vi "Traverse Folder.vi"(5 "NEXT":bool, 7 "PREV":bool, 8 "error in (no error)":errorcluster, 10 "Context":T1, 11 "Boolean in":refnum<vi>) -> (0 "error out":errorcluster, 2 "Context out":T1)   [LabVIEW 2020, in "DocTool.lvlib"]
uses:
  DocTool.lvlib
  TDefs/Context.ctl
  Events.ctl
  UserEvent.ctl
  TDefs/State.ctl
  TDefs/States.ctl
  TDefs/Single File Properties.ctl
  TDefs/FP Items Properties.ctl
  TDefs/FP Item Properties.ctl
  TDefs/CopyTag.ctl
  d44677d1-7ccb-46bd-9aaf-ca2af3999deb.vi
  StateMachine.lvlib
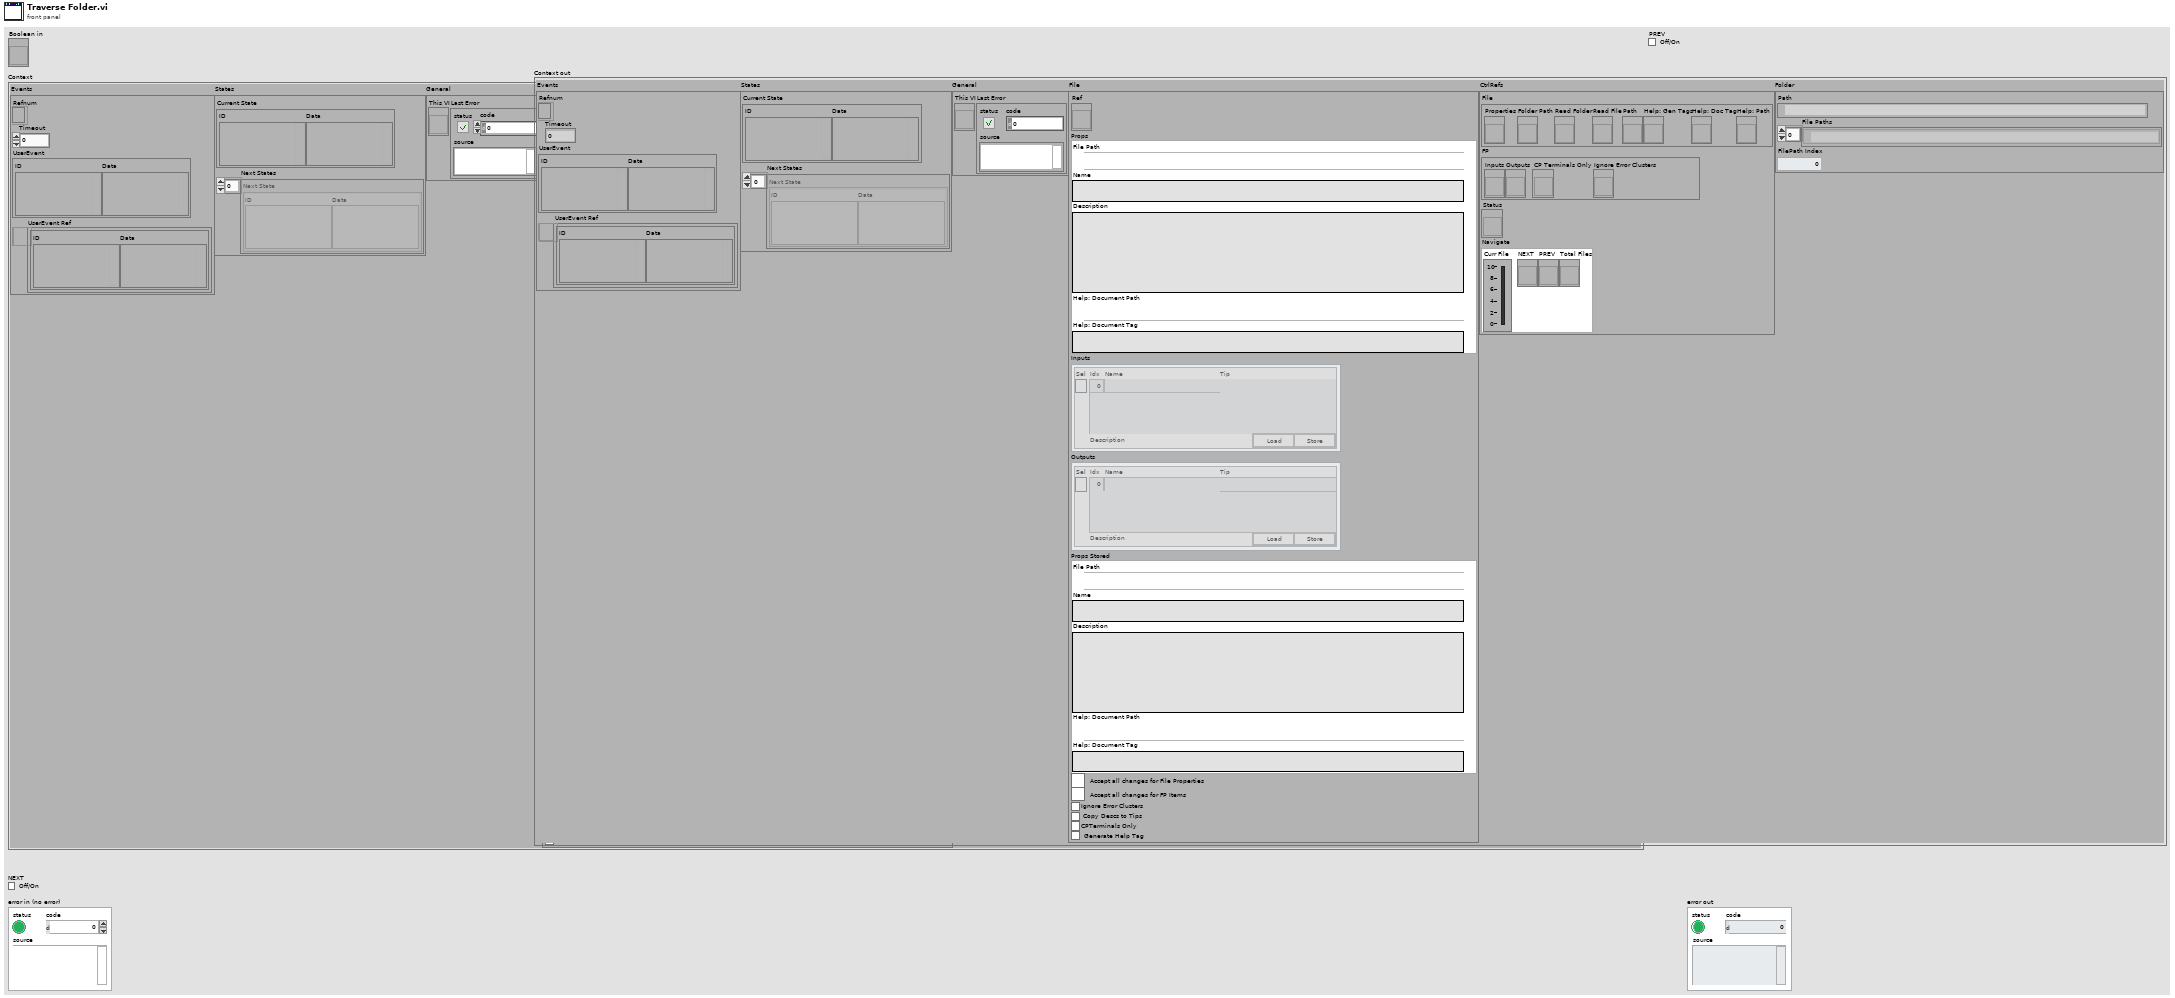
[diagram p1: front panel]
types:
  T1 = typedef "DocTool.lvlib/Context.ctl" = cluster{"Events":T2, "States":cluster{"Current State":T4, "Next States":T5}, "General":cluster{"This VI":refnum<vi>, "Last Error":errorcluster}, "File":cluster{"Ref":refnum<vi>, "Props":T6, "Inputs":T7, "Outputs":T7, "Props Stored":T6, "Write":bool, "Write FP":bool, "Ignore Error Clusters":bool, "Copy Descs to Tips":bool, "CPTerminals Only":bool, "Generate Help Tag":bool}, "CtrlRefs":cluster{"File":cluster{"Properties":refnum<vi>, "Folder Path":refnum<vi>, "Read Folder":refnum<vi>, "Read File":refnum<vi>, "Path":refnum<vi>, "Help: Gen Tags":refnum<vi>, "Help: Doc Tag":refnum<vi>, "Help: Path":refnum<vi>}, "FP":cluster{"Inputs":refnum<vi>, "Outputs":refnum<vi>, "CP Terminals Only":refnum<vi>, "Ignore Error Clusters":refnum<vi>}, "Status":refnum<vi>, "Navigate":cluster{"Curr File":refnum<vi>, "NEXT":refnum<vi>, "PREV":refnum<vi>, "Total Files":refnum<vi>}}, "Folder":cluster{"Path":path, "File Paths":path[], "FilePath Index":i32}}
  T2 = typedef "StateMachine.lvlib/Events.ctl" = cluster{"Refnum":refnum<event-registration>, "Timeout":i32, "UserEvent":T3, "UserEvent Ref":refnum<user-event>}
  T3 = typedef "StateMachine.lvlib/UserEvent.ctl" = cluster{"ID":variant, "Data":variant}
  T4 = typedef "StateMachine.lvlib/State.ctl" = cluster{"ID":variant, "Data":variant}
  T5 = typedef "StateMachine.lvlib/States.ctl" = T4[]
  T6 = typedef "DocTool.lvlib/Single File Properties.ctl" = cluster{"File Path":path, "Name":string, "Description":string, "Help: Document Path":path, "Help: Document Tag":string}
  T7 = typedef "DocTool.lvlib/FP Items Properties.ctl" = T8[]
  T8 = typedef "DocTool.lvlib/FP Item Properties.ctl" = cluster{"Sel":bool, "Idx":i32, "Name":string, "Description":string, "Tip":string, "Load Store":T9}
  T9 = typedef "DocTool.lvlib/CopyTag.ctl" = cluster{"Load":bool, "Store":bool}
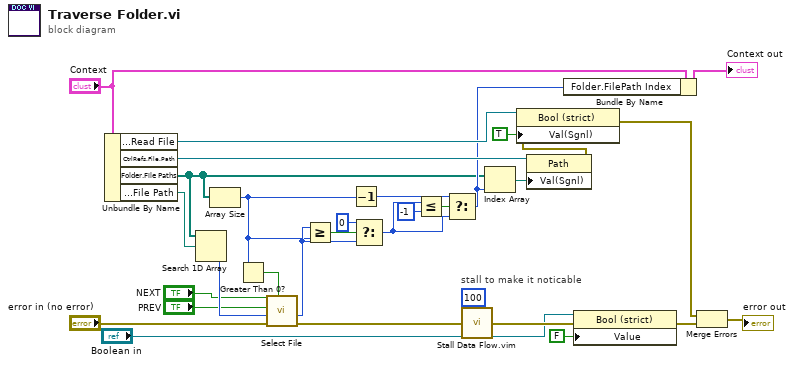
[diagram p0: block diagram]
diagram:
  # "stall to make it noticable"
  n1 = Unbundle By Name("Context") -> ("CtrlRefs.File.Read File"=w28:refnum<vi>, "CtrlRefs.File.Path"=w25:refnum<vi>, "Folder.File Paths"=w2:path[], "File.Props.File Path"=w26:path)
  n2 = Search 1D Array(1D array=w2, element=w26) -> (index of element=w27:i32)  [unwired: 1 in]
  n3 = Array Size(array=w2) -> (size(s)=w3:i32)
  n4 = Greater Than 0?(x=w3) -> (x > 0?=w6:bool)
  n5 = call "Select File.vi"("Files Found"=w6, "error in (no error)"="error in (no error)", "Current File in"=w27, "PREV"="PREV", "NEXT"="NEXT") -> ("error out"=w12:errorcluster, "Current File out"=w23:i32)  [unwired: 5 in]
  n6 = Greater Or Equal?(x=w23, y=w3) -> (x >= y?=w17:bool)
  n7 = Decrement(x=w3) -> (x-1=w21:i32)
  n8 = Select(t=0, s=w17, f=w23) -> (s? t:f=w22:i32)
  n9 = Less Or Equal?(x=w22, y=-1) -> (x <= y?=w20:bool)
  n10 = Select(t=w21, s=w20, f=w22) -> (s? t:f=w4:i32)
  n11 = call "Stall Data Flow.vim"("value in"=w12, "milliseconds to wait"=u32 100) -> ("value out"=w15:errorcluster)  [unwired: 1 out]
  n12 = Index Array(array=w2, index=w4) -> (element=w24:path)
  n13 = property class="Path"(reference=w25, "Val(Sgnl)"=w24) -> (error out=w30:errorcluster)  [unwired: 1 in, 1 out]
  n14 = property class="Bool (strict)"(reference=w28, error in=w30, "Val(Sgnl)"=TRUE ("Value (Signaling)")) -> (error out=w1:errorcluster)  [unwired: 1 out]
  n15 = Bundle By Name(cluster="Context", "Folder.FilePath Index"=w4) -> (→"Context out":T1)
  n16 = property class="Bool (strict)"(reference="Boolean in", error in=w15, "Value"=FALSE) -> (error out=w13:errorcluster)  [unwired: 1 out]
  n17 = Merge Errors(w1, w13) -> (→"error out":errorcluster)
